vi "Actor Core.vi"(8 "error in":errorcluster, 11 "LeakyViewable In":refnum<class "LeakyViewable.lvclass">) -> (0 "error out":errorcluster, 3 "Actor out":refnum<class "Actor.lvclass">)   [LabVIEW 2017, in "ViewableDoubles.lvlib" / "LeakyViewable.lvclass"]
doc: "(<B>Filename</B>: Actor Framework.lvlib:Actor.lvclass:Actor Core.vi)\n\nReceives messages to the actor, reacts to them, and initiates any error handling that may shut the actor down.\n\nDescendant classes may override this VI to append parallel tasks for the actor to complete while it handles messages. Overrides use the Call Parent Method node.\n\n<License>\nCopyright © 2017 Composed Systems, LLC | All rights reserved\nwww.composed.io\n\nAuthor: Ethan Stern <ethan.stern@composed.io>\n\nThis software is provided \"AS IS\" WITHOUT WARRANTIES, either express or implied, AND IS FOR EDUCATIONAL PURPOSES ONLY.\n</License>"
uses:
  LeakyViewable.lvclass
  LeakyViewable Messages/Leak Viewable State Msg/Leak Viewable State Msg.lvclass
  <vilib>/ActorFramework/Actor/Actor.lvclass
  <vilib>/ActorFramework/Message Enqueuer/Message Priority.ctl
  <vilib>/ActorFramework/Message Enqueuer/Message Enqueuer.lvclass
  gpm_packages/@cs/mva-viewable/Source/IViewable/IViewable/IViewable.lvclass
  Leak Location.ctl
  C:/Program Files (x86)/National Instruments/LabVIEW 2017/vi.lib/ActorFramework/Actor/Actor.lvclass
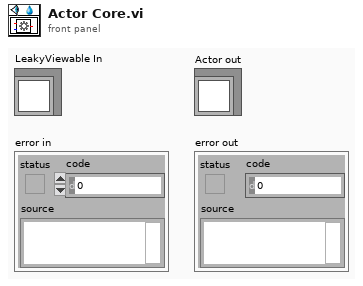
[diagram p1: front panel]
types:
  T1 = typedef "ViewableDoubles.lvlib/LeakyViewable.lvclass/Leak Location.ctl" = enum16{"Pre Launch Init", "Entering Actor Core", "Actor Core", "Exiting Actor Core", "Stop Core", "Handle Error"}
  T2 = typedef "Actor Framework.lvlib/Message Enqueuer.lvclass/Message Priority.ctl" = enum16{"Low", "Normal", "High"}
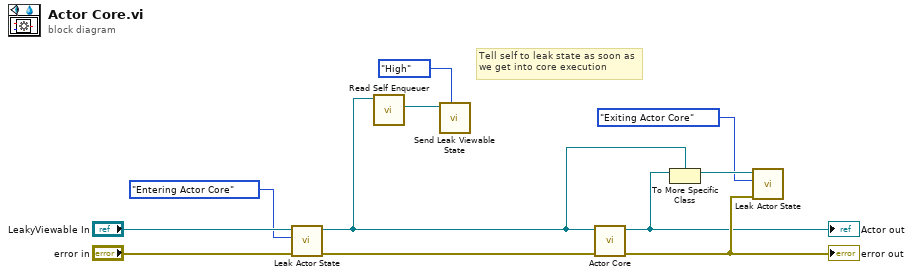
[diagram p0: block diagram]
diagram:
  # "Tell self to leak state as soon as\nwe get into core execution"
  n1 = call "Leak Actor State.vi"("error in (no error)"="error in", "Location"=Leak_Location."Entering Actor Core", "ViewableOne in"="LeakyViewable In") -> ("error out"=w8:errorcluster, "ViewableOne out"=w3:refnum<class "LeakyViewable.lvclass">)  [unwired: 7 in]
  n2 = call <vilib>:"Read Self Enqueuer.vi"("Actor"=w3) -> ("Self Enqueuer"=w10:refnum<class "Message Enqueuer.lvclass">)  [unwired: 10 in]
  n3 = call "Send Leak Viewable State.vi"("Message Priority (Normal)"=Message_Priority."High", "Message Enqueuer"=w10) -> ()  [unwired: 8 in, 2 out]
  n4 = call-parent "Actor Core.vi"("error in"=w8, "IViewable In"=w3) -> ("error out"=w6:errorcluster, "Actor out"=w5:refnum<class "Actor.lvclass">)  [unwired: 8 in]
  "error out" <- w6
  "Actor out" <- w5
  n5 = To More Specific Class(target class=w3, reference=w5) -> (specific class reference=w4:refnum<class "LeakyViewable.lvclass">)  [unwired: 1 in, 1 out]
  n6 = call "Leak Actor State.vi"("error in (no error)"=w6, "Location"=Leak_Location."Exiting Actor Core", "ViewableOne in"=w4) -> ()  [unwired: 7 in, 2 out]
